vi "Tatrocki_B_2.vi"   [LabVIEW 2020]
uses:
  <vilib>/Platform/TimedLoop/XDataNode/timing_clust.ctl
  <vilib>/Platform/TimedLoop/XDataNode/nitl_modes.ctl
  <vilib>/Platform/TimedLoop/XDataNode/wakeup.ctl
  <vilib>/platform/TimedLoop/XDataNode/XDataNode.xnode
  <vilib>/Platform/TimedLoop/XDataNode/XDNodeRunTimeDep.lvlib
types:
  T1 = typedef "Rendezvous RefNum" = refnum<k1>
  T2 = typedef "XDNodeRunTimeDep.lvlib/timing_clust.ctl" = cluster{"Expected End [f-1]":u64, "Actual End [f-1]":u64, "Finished Late? [f-1]":bool, "Expected End [i-1]":u64, "Actual End [i-1]":u64, "Finished Late? [i-1]":bool, "Expected Start [i]":u64, "Actual Start [i]":u64, "Expected Start [f]":u64, "Actual Start [f]":u64, "Source Name":string, "Structure Name":string, "Period":i64, "Deadline":i64, "Offset":i64, "Start":i64, "Priority":i32, "Timeout":i32, "Mode":T3, "Wakeup Reason":T4, "Error":errorcluster, "Source Type":string, "Secondary Source Type":string, "Global End Time":u64, "Global Start Time":u64, "Frame Duration":u64, "Iteration Duration":u64, "Assigned CPU":i32, "I/O Scan Engine Mode":u32}
  T3 = typedef "XDNodeRunTimeDep.lvlib/nitl_modes.ctl" = enum32{"No Change", "Process missed periods, maintain original phase", "Discard missed periods, maintain original phase", "Process missed periods, ignore original phase", "Discard missed periods, ignore original phase"}
  T4 = typedef "XDNodeRunTimeDep.lvlib/wakeup.ctl" = enum32{"Normal", "Aborted", "Asynchronous wakeup", "Timing source error", "Timed loop error", "Timeout"}
  T5 = typedef "Semaphore RefNum" = refnum<k1>
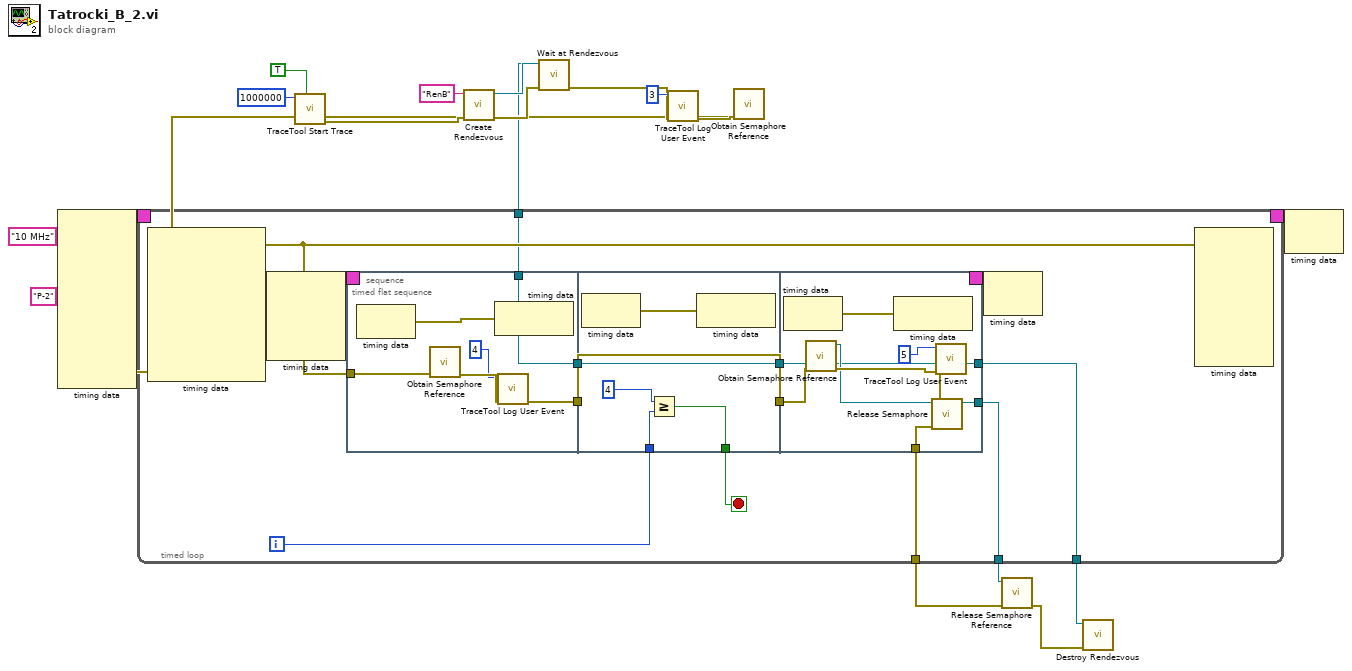
[diagram p0: block diagram]
diagram:
  n1 = call <vilib>:"TraceTool Start Trace.vi"("Detailed Tracing? (F)"=TRUE, "Buffer Size (250000 bytes)"=1000000) -> ("error out"=w14:errorcluster)  [unwired: 8 in, 1 out]
  n2 = call <vilib>:"Create Rendezvous.vi"("error in (no error)"=w14, "name (unnamed)"="RenB") -> ("error out"=w13:errorcluster, "rendezvous"=w16:T1)  [unwired: 3 in, 1 out]
  n3 = call <vilib>:"Wait at Rendezvous.vi"("error in (no error)"=w13, "rendezvous"=w16) -> ("error out"=w12:errorcluster, "rendezvous out"=w2:T1)  [unwired: 3 in, 1 out]
  n4 = call <vilib>:"TraceTool Log User Event.vi"("error in (no error)"=w12, "Event ID (0-255)"=u32 3) -> ("error out"=w11:errorcluster)  [unwired: 9 in]
  n5 = call <vilib>:"Obtain Semaphore Reference.vi"("error in (no error)"=w11) -> ("error out"=w6:errorcluster)  [unwired: 4 in, 2 out]
  n6 = node-c288("10 MHz" ("Source Name"), "P-2" ("Structure Name"), w6) -> (w10:T2)  [unwired: 7 in]
  n7 = timed-loop {
    timing: w10 -> [_]
    timing-out: [_] -> w9
    tunnel: [w23] -> w5
    tunnel: [w22] -> w3
    tunnel: w2 -> [w21]
    tunnel: [w20] -> w1
    i -> [w26]
    stop <- w25 stop-if-true
    n8 = node-c288() -> (w24:errorcluster)  [unwired: 1 in, 8 out]
    n9 = node-c288() -> (w28:T2)  [unwired: 4 in]
    n10 = timed-sequence {
      timing: w28 -> [_]
      timing-out: [_] -> w27
      tunnel: w26 -> [w39]
      tunnel: [w38] -> w25
      tunnel: w24 -> [w37]
      tunnel: [w34] -> w23
      tunnel: [w33] -> w22
      tunnel: w21 -> [w31]
      tunnel: [w30] -> w20
      n11 = timed-flat-sequence {
        tunnel: w37 -> [w42]
        tunnel: [w41] -> w35
        tunnel: [w40] -> w32
        tunnel: w31 -> [w40]
        tunnel: w39 -> [w55]
        tunnel: [w54] -> w38
        tunnel: [w53] -> w36
        tunnel: w35 -> [w53]
        tunnel: w32 -> [w51]
        tunnel: [w51] -> w29
        tunnel: w36 -> [w65]
        tunnel: [w66] -> w34
        tunnel: [w63] -> w33
        tunnel: [w62] -> w30
        tunnel: w29 -> [w62]
        frame #0 {
          n12 = node-c288() -> (w45:errorcluster)  [unwired: 1 in]
          n13 = call <vilib>:"Obtain Semaphore Reference.vi"("error in (no error)"=w42) -> ("error out"=w44:errorcluster)  [unwired: 4 in, 2 out]
          n14 = node-c288(w45) -> ()  [unwired: 1 out]
          n15 = call <vilib>:"TraceTool Log User Event.vi"("error in (no error)"=w44, "Event ID (0-255)"=u32 4) -> ("error out"=w41:errorcluster)  [unwired: 9 in]
        }
        frame #1 {
          n16 = node-c288() -> (w56:errorcluster)  [unwired: 1 in]
          n17 = Greater Or Equal?(x=4, y=w55) -> (x >= y?=w54:bool)
          n18 = node-c288(w56) -> ()  [unwired: 1 out]
        }
        frame #2 {
          n19 = node-c288() -> (w70:errorcluster)  [unwired: 1 in]
          n20 = call <vilib>:"Obtain Semaphore Reference.vi"("error in (no error)"=w65) -> ("error out"=w69:errorcluster, "semaphore"=w64:T5)  [unwired: 4 in, 1 out]
          n21 = node-c288(w70) -> ()  [unwired: 1 out]
          n22 = call <vilib>:"TraceTool Log User Event.vi"("error in (no error)"=w69, "Event ID (0-255)"=u32 5) -> ("error out"=w67:errorcluster)  [unwired: 9 in]
          n23 = call <vilib>:"Release Semaphore.vi"("error in (no error)"=w67, "semaphore"=w64) -> ("error out"=w66:errorcluster, "semaphore out"=w63:T5)  [unwired: 4 in]
        }
      }
    }
    n24 = node-c288(w27) -> ()  [unwired: 1 out]
    n25 = node-c288(w24) -> ()  [unwired: 7 in, 1 out]
  }
  n26 = call <vilib>:"Release Semaphore Reference.vi"("error in (no error)"=w5, "semaphore"=w3) -> ("error out"=w4:errorcluster)  [unwired: 8 in, 1 out]
  n27 = call <vilib>:"Destroy Rendezvous.vi"("error in (no error)"=w4, "rendezvous"=w1) -> ()  [unwired: 4 in, 2 out]
  n28 = node-c288(w9) -> ()  [unwired: 1 out]
